vi "RSZVB Modify Source Power Calibration Settings.vi"(0 "VISA session":refnum<visa-resource-name>, 1 "Channel (1)":i32=1, 2 "Port Number (1)":i32=1, 3 "Number Of Readings (1)":i32=1, 4 "Tolerance (1)":dbl=1.0 format="%^.3e", 5 "error in (no error)":errorcluster {"code" format="%.0x"}, 6 "Port Power Offset (0)":dbl format="%^.3e", 7 "Offset Parameter (1: Add Channel Power)":i32(ring)=1 items=["Only", "Add Channel Power"], 8 "Calibration Power Offset (0)":dbl format="%^.3e", 9 "Other Sources (T: On)":bool=TRUE) -> (14 "dup VISA session":refnum<visa-resource-name>, 19 "error out":errorcluster {"code" format="%.0x"})   [LabVIEW 2011]
doc: "This VI configures the source power calibration settings\n\nRemote-control command(s):\nSOURce<Ch>:POWer<Pt>:CORRection:NREadings <readings>\nSOURce<Ch>:POWer<Pt>:CORRection:COLLect:AVERage:NTOLerance <tolerance>\nSOURce<Ch>:POWer<Pt>:CORRection:OSOurces[:STATe] ON | OFF \nSOURce<Ch>:POWer<Pt>[:LEVel][:IMMediate]:OFFSet <numeric_value>, ONLY | CPADd\nSOURce<Ch>:POWer<Pt>:CORRection:LEVel:OFFSet <numeric_value>"
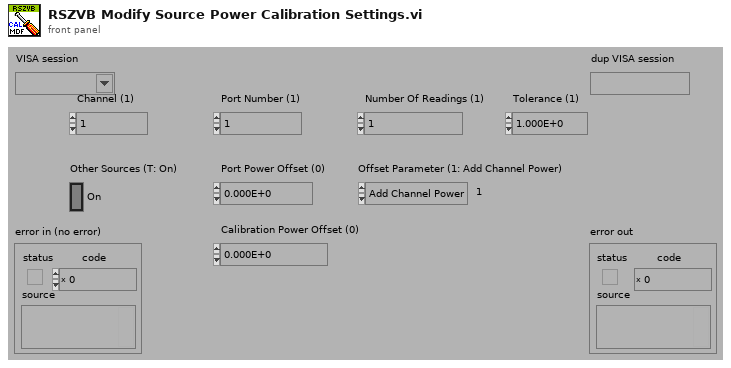
[diagram p1: front panel]
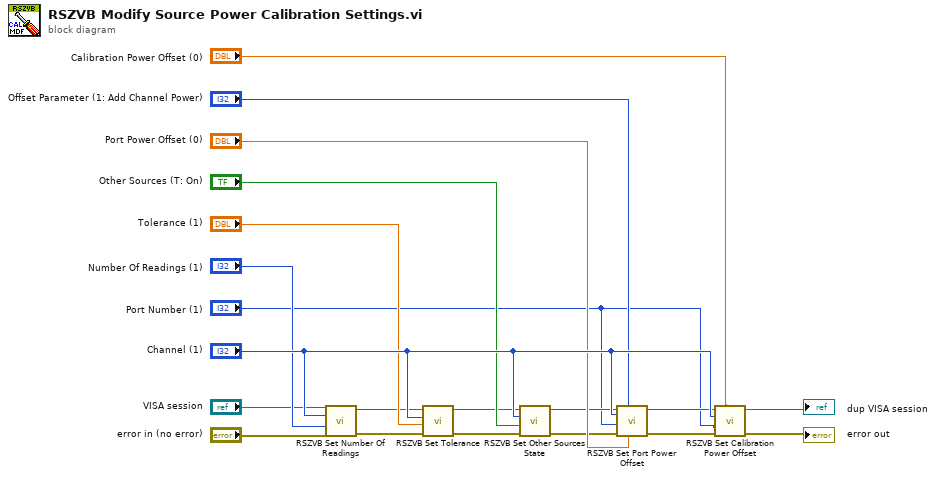
[diagram p0: block diagram]
diagram:
  n1 = call "RSZVB Set Number Of Readings.vi"("error in (no error)"="error in (no error)", "Number Of Readings (1)"="Number Of Readings (1)", "Channel (1)"="Channel (1)", "VISA session"="VISA session") -> ("error out"=w7:errorcluster, "dup VISA session"=w13:refnum<visa-resource-name>)  [unwired: 6 in]
  n2 = call "RSZVB Set Tolerance.vi"("error in (no error)"=w7, "Tolerance (1.0)"="Tolerance (1)", "Channel (1)"="Channel (1)", "VISA session"=w13) -> ("error out"=w6:errorcluster, "dup VISA session"=w12:refnum<visa-resource-name>)  [unwired: 6 in]
  n3 = call "RSZVB Set Other Sources State.vi"("error in (no error)"=w6, "Other Sources (T: On)"="Other Sources (T: On)", "Channel (1)"="Channel (1)", "VISA session"=w12) -> ("error out"=w5:errorcluster, "dup VISA session"=w11:refnum<visa-resource-name>)  [unwired: 6 in]
  n4 = call "RSZVB Set Port Power Offset.vi"("Port Power Offset (0)"="Port Power Offset (0)", "Offset Parameter (1: Add Channel Power)"="Offset Parameter (1: Add Channel Power)", "error in (no error)"=w5, "Port Number (1)"="Port Number (1)", "Channel (1)"="Channel (1)", "VISA session"=w11) -> ("error out"=w4:errorcluster, "dup VISA session"=w10:refnum<visa-resource-name>)  [unwired: 4 in]
  n5 = call "RSZVB Set Calibration Power Offset.vi"("Calibration Power Offset (0)"="Calibration Power Offset (0)", "error in (no error)"=w4, "Port Number (1)"="Port Number (1)", "Channel (1)"="Channel (1)", "VISA session"=w10) -> ("error out"=→"error out":errorcluster, "dup VISA session"=→"dup VISA session":refnum<visa-resource-name>)  [unwired: 5 in]
